vi "Create Dialog Actor.vi"(4 "Calling VI Ref":refnum<vi>, 5 "Bar Visibility":T1={"Menu Bar"=FALSE, "Title Bar"=TRUE}, 6 "Launch Position (Centered)":T3=enum."Centered", 7 "Scrollbars (off)":T2, 8 "error in (no error)":errorcluster, 9 "Dialog Behavior":T4(ring)=enum."Default", 10 "UI VI Reference (caller)":refnum<vi>, 11 "Flex  Dialog (Actor) in":refnum<class "Flex Dialog (Actor).lvclass">) -> (0 "error out":errorcluster, 3 "Flex  Dialog (Actor) out":refnum<class "Flex Dialog (Actor).lvclass">)   [LabVIEW 2016, in "Flex UI Dialog (Actor).lvlib" / "Flex Dialog (Actor).lvclass"]
uses:
  Flex Dialog (Actor).lvclass
  <vilib>/East West Architects/Flex UI/Flex UI Dialog/Enum - Launch Position.ctl
  <vilib>/East West Architects/Flex UI/Flex UI Dialog/Cluster - Scrollbar Settings.ctl
  <vilib>/East West Architects/Flex UI/Flex UI Dialog/Cluster - Bar Visibility.ctl
  <vilib>/East West Architects/Flex UI/Flex UI Dialog/Flex UI Dialog.lvclass
  C:/Program Files (x86)/National Instruments/LabVIEW 2016/vi.lib/East West Architects/Flex UI/Flex UI (Parent)/Flex UI.lvclass
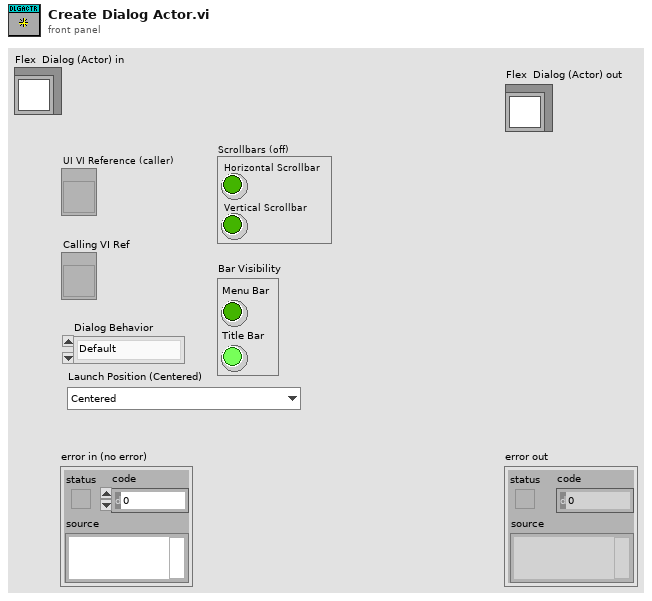
[diagram p1: front panel]
types:
  T1 = typedef "Flex UI Dialog.lvclass/Cluster - Bar Visibility.ctl" = cluster{"Menu Bar":bool, "Title Bar":bool}
  T2 = typedef "Flex UI Dialog.lvclass/Cluster - Scrollbar Settings.ctl" = cluster{"Horizontal Scrollbar":bool, "Vertical Scrollbar":bool}
  T3 = typedef "Flex UI Dialog.lvclass/Enum - Launch Position.ctl" = enum16{"Default (Last Opened)", "Centered", "Centered on Caller", "Maximized", "Hidden"}
  T4 = enum32{"Invalid", "Default", "Floating", "Floating/Auto-Hide", "Modal"}
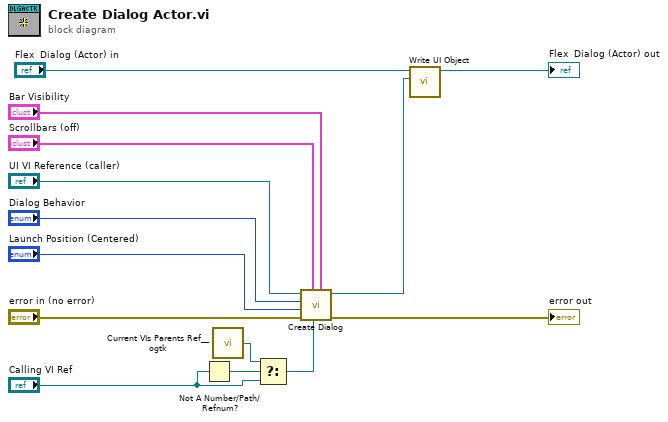
[diagram p0: block diagram]
diagram:
  n1 = Not A Number/Path/Refnum?(number/path/refnum="Calling VI Ref") -> (NaN/Path/Refnum?=w4:bool)
  n2 = call <userlib>:"Current VIs Parents Ref__ogtk.vi"() -> ("Calling VI's Reference"=w3:refnum<vi>)  [unwired: 2 in]
  n3 = Select(t=w3, s=w4, f="Calling VI Ref") -> (s? t:f=w2:refnum<vi>)
  n4 = call <vilib>:"Create Dialog.vi"("Bar Visibility"="Bar Visibility", "Calling VI Reference"=w2, "Scrollbars (off)"="Scrollbars (off)", "error in"="error in (no error)", "Launch Position (Centered)"="Launch Position (Centered)", "Dialog Behavior"="Dialog Behavior", "UI VI Reference (caller)"="UI VI Reference (caller)") -> ("error out"=→"error out":errorcluster, "Flex Dialog out"=w1:refnum<class "Flex UI Dialog.lvclass">)  [unwired: 3 in]
  n5 = call-dynamic "Write UI Object.vi"("Flex UI in"=w1, "Flex UI (Actor) in"="Flex  Dialog (Actor) in") -> ("Flex UI (Actor) out"=→"Flex  Dialog (Actor) out":refnum<class "Flex Dialog (Actor).lvclass">)  [unwired: 8 in, 1 out]
